vi "VII Init I2C.vi"(7 "pInitConfig":T1, 8 "error in (no error)":errorcluster, 9 "I2CIndex":i32, 10 "DevIndex":i32, 11 "DevType":i32) -> (0 "error out":errorcluster, 3 "function return":i32)   [LabVIEW 2012, in "ControlI2C.lvlib"]
doc: "int __stdcall VII_InitI2C(int DevType, int DevIndex, int I2CIndex, PVII_INIT_CONFIG pInitConfig);"
uses:
  ControlI2C.lvlib
  Ginkgo_Driver.dll
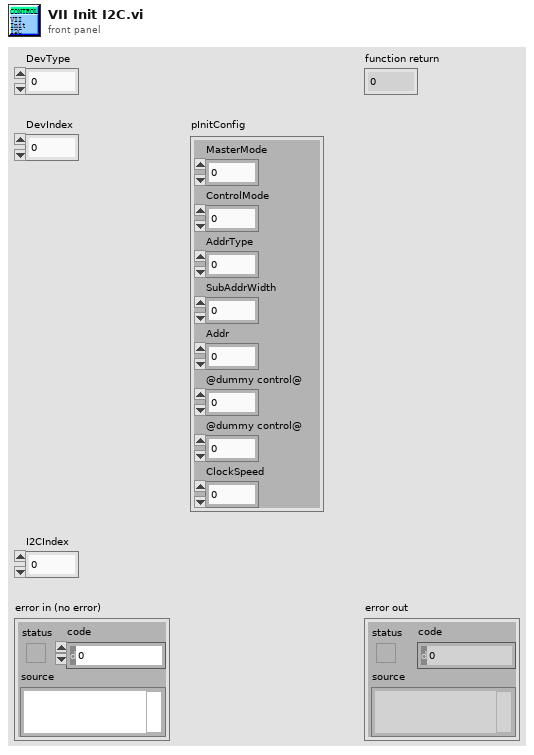
[diagram p1: front panel]
types:
  T1 = cluster{"MasterMode":u8, "ControlMode":u8, "AddrType":u8, "SubAddrWidth":u8, "Addr":u16, "@dummy control@":i8, "@dummy control@":i8, "ClockSpeed":i32}
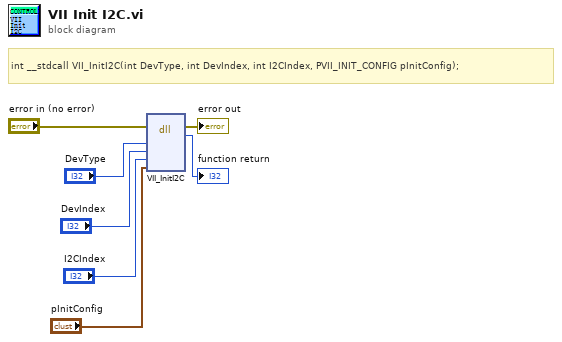
[diagram p0: block diagram]
diagram:
  # "int __stdcall VII_InitI2C(int DevType, int DevIndex, int I2CIndex, PVII_INIT_CONFIG pInitConfig);"
  n1 = dll-call lib="E:/Project/vt_ginkgo/truck/Ginkgo Driver/vs2010/Ginkgo_USB-I2C_API_v2.0.3.0/lib/labview_32bit/ControlI2C/Ginkgo_Driver.*" fn="VII_InitI2C"(error in="error in (no error)", "DevType"="DevType", "DevIndex"="DevIndex", "I2CIndex"="I2CIndex", "pInitConfig"="pInitConfig") -> (error out=→"error out":errorcluster, →"function return":i32)  [unwired: 6 in, 1 out]
